vi "Config_displayGeneral.vi"(8 "error in (no error)":errorcluster, 10 "Config Data":T1, 11 "Cluster in":refnum<vi>) -> (0 "error out":errorcluster)   [LabVIEW 2014]
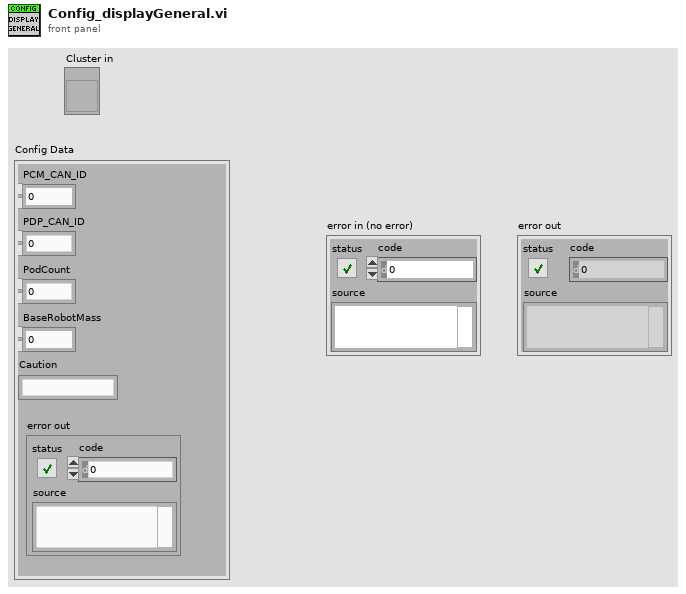
[diagram p1: front panel]
types:
  T1 = cluster{"PCM_CAN_ID":dbl, "PDP_CAN_ID":dbl, "PodCount":dbl, "BaseRobotMass":dbl, "Caution":string, "error out":errorcluster}
  T2 = cluster{"PCM_CAN_ID":dbl, "PDP_CAN_ID":dbl, "PodCount":dbl, "BaseRobotMass":dbl, "Caution":string}
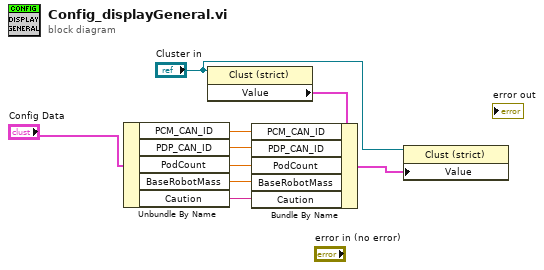
[diagram p0: block diagram]
diagram:
  n1 = Unbundle By Name("Config Data") -> ("PCM_CAN_ID"=w7:dbl, "PDP_CAN_ID"=w6:dbl, "PodCount"=w5:dbl, "BaseRobotMass"=w4:dbl, "Caution"=w3:string)
  n2 = property class="Clust (strict)"(reference="Cluster in") -> ("Value"=w8:T2)  [unwired: 1 in, 2 out]
  n3 = Bundle By Name(cluster=w8, "PCM_CAN_ID"=w7, "PDP_CAN_ID"=w6, "PodCount"=w5, "BaseRobotMass"=w4, "Caution"=w3) -> (w9:T2)
  n4 = property class="Clust (strict)"(reference="Cluster in", "Value"=w9) -> ()  [unwired: 1 in, 2 out]
